vi "m1m3_getNextSample_HardpointActuatorData.vi"(8 "error in (no error)":errorcluster, 11 "HardpointActuatorData_Ctl":T1={"Timestamp"=0.0, "StepsQueued[6]"=[0, 0, 0, 0, 0, 0], "StepsCommanded[6]"=[0, 0, 0, 0, 0, 0], "MeasuredForce[6]"=[0.0, 0.0, 0.0, 0.0, 0.0, 0.0], "Encoder[6]"=[0, 0, 0, 0, 0, 0], "Displacement[6]"=[0.0, 0.0, 0.0, 0.0, 0.0, 0.0], "Fx"=0.0, "Fy"=0.0, "Fz"=0.0, "Mx"=0.0, "My"=0.0, "Mz"=0.0, "ForceMagnitude"=0.0, "XPosition"=0.0, "YPosition"=0.0, "ZPosition"=0.0, "XRotation"=0.0, "YRotation"=0.0, "ZRotation"=0.0}) -> (0 "error out":errorcluster, 2 "function return":i32, 3 "HardpointActuatorData_Ctl out":T1)   [LabVIEW 2016, in "SALLV_m1m3.lvlib"]
doc: "int m1m3_shm_getNextSample_HardpointActuatorDataLV(m1m3_HardpointActuatorDataLV *HardpointActuatorData_Ctl );"
uses:
  SALLV_m1m3.lvlib
  DataTypes/HardpointActuatorData.ctl
  SALLV_m1m3.so
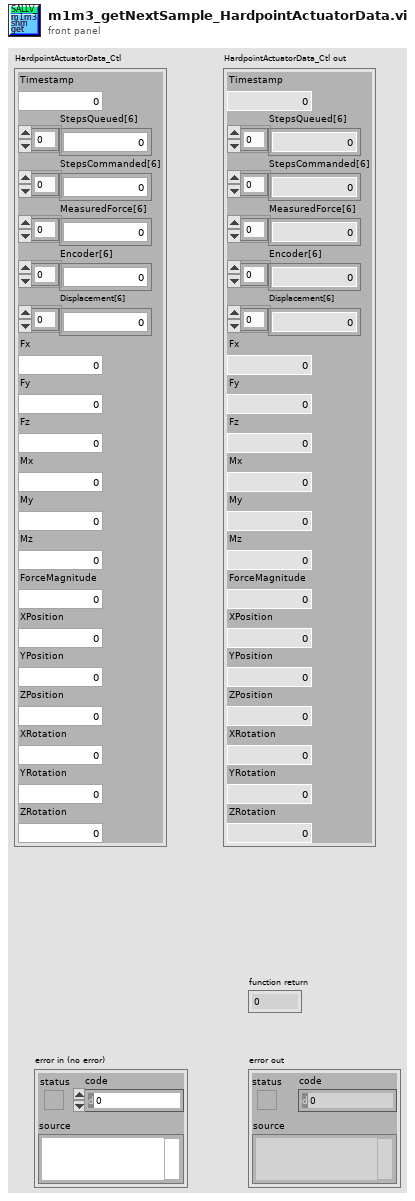
[diagram p1: front panel]
types:
  T1 = typedef "SALLV_m1m3.lvlib/HardpointActuatorData.ctl" = cluster{"Timestamp":dbl, "StepsQueued[6]":i32[], "StepsCommanded[6]":i16[], "MeasuredForce[6]":sgl[], "Encoder[6]":i32[], "Displacement[6]":sgl[], "Fx":sgl, "Fy":sgl, "Fz":sgl, "Mx":sgl, "My":sgl, "Mz":sgl, "ForceMagnitude":sgl, "XPosition":sgl, "YPosition":sgl, "ZPosition":sgl, "XRotation":sgl, "YRotation":sgl, "ZRotation":sgl}
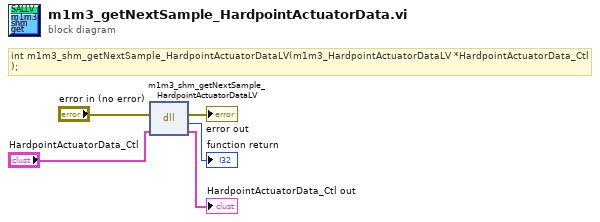
[diagram p0: block diagram]
diagram:
  # "int m1m3_shm_getNextSample_HardpointActuatorDataLV(m1m3_HardpointActuatorDataLV *HardpointActuatorData_Ctl );"
  n1 = dll-call lib="opt/CODE/SALLV_m1m3/SALLV_m1m3.*" fn="m1m3_shm_getNextSample_HardpointActuatorDataLV"(error in="error in (no error)", "HardpointActuatorData_Ctl"="HardpointActuatorData_Ctl") -> (error out=→"error out":errorcluster, →"function return":i32, "HardpointActuatorData_Ctl"=→"HardpointActuatorData_Ctl out":T1)  [unwired: 2 in, 1 out]
